vi "AUTON_Index.vi"(0 "Auton Array":dbl[][](array[numeric]), 5 "MeasuredHeading":dbl, 7 "LeftEncoder":dbl, 9 "RightEncoder":dbl) -> (4 "Right Drive":dbl, 6 "Left Drive":dbl, 8 "Harvester":dbl, 10 "Winch":dbl, 15 "Cam":dbl)   [LabVIEW 2013]
uses:
  Robot Global Data.vi
panel:
  in  "BallOnShooter":bool
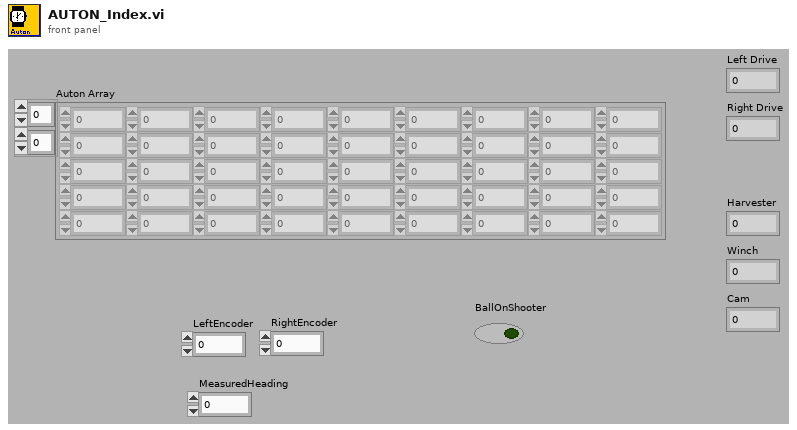
[diagram p1: front panel]
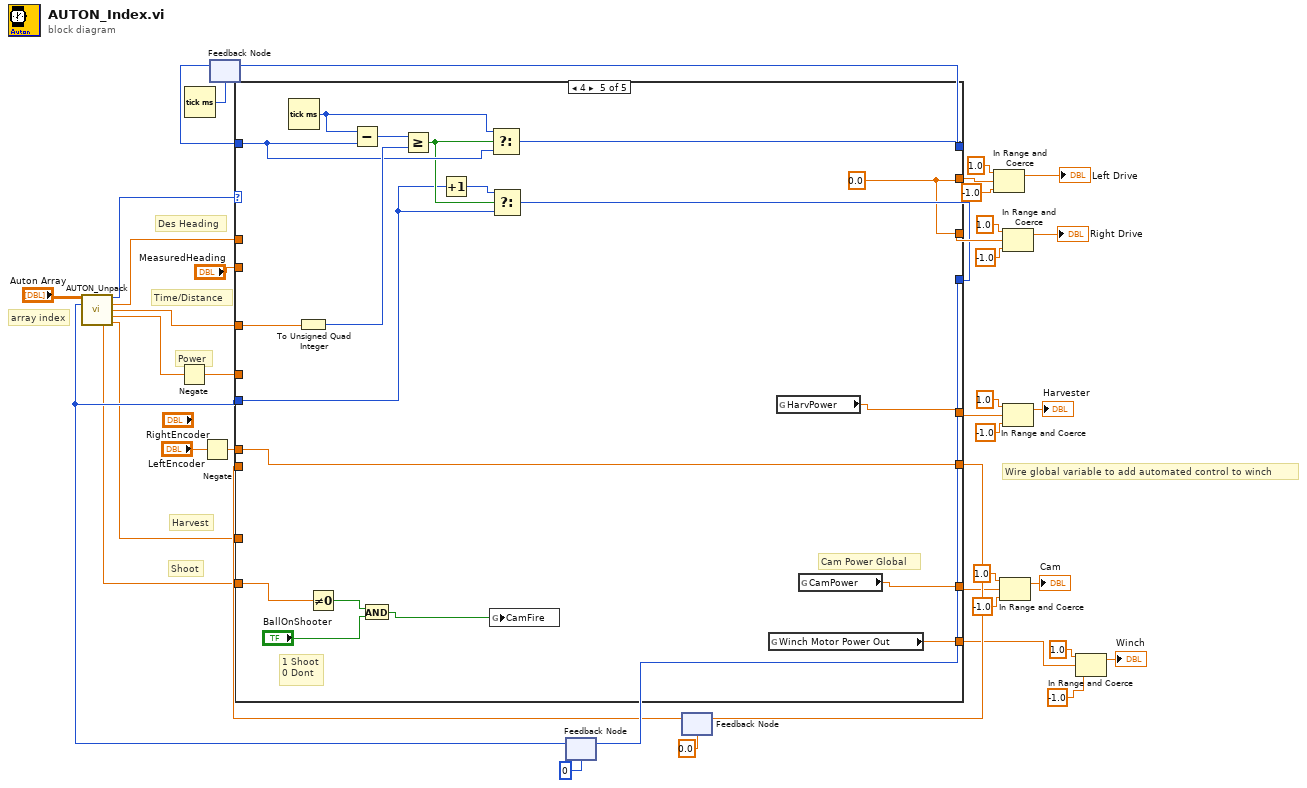
[diagram p0: block diagram]
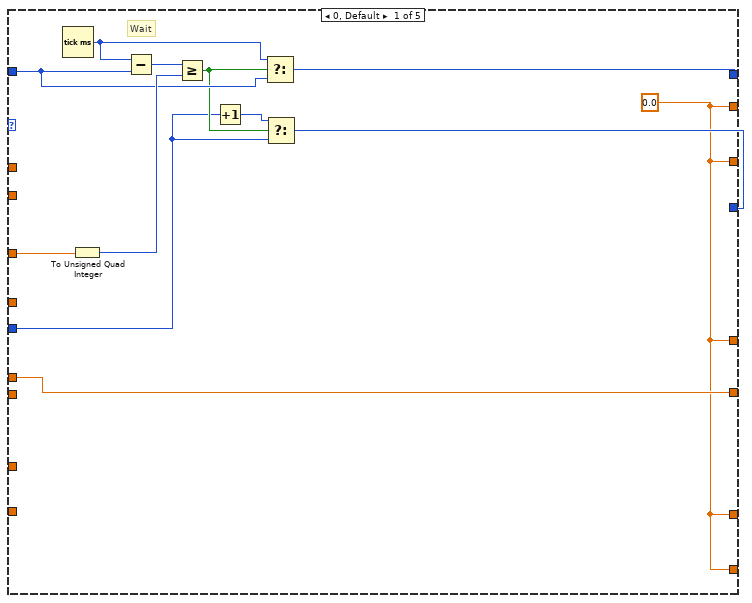
[diagram p2: hidden frame]
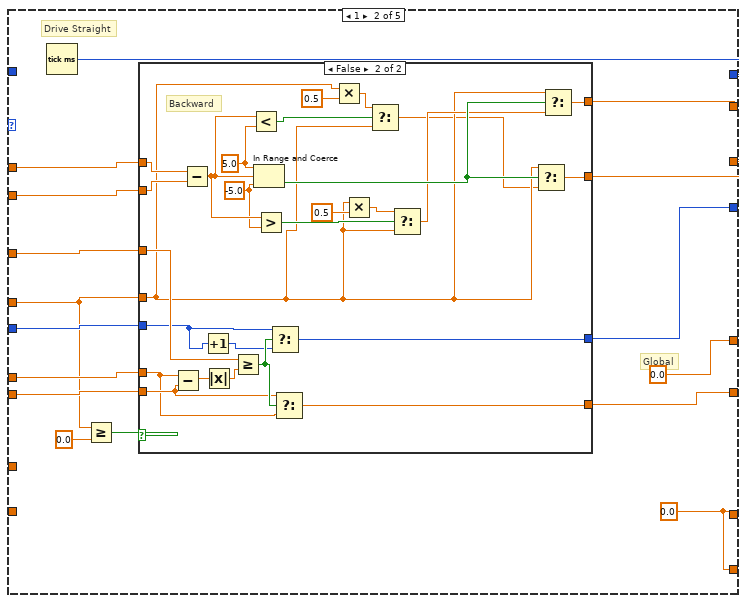
[diagram p3: hidden frame]
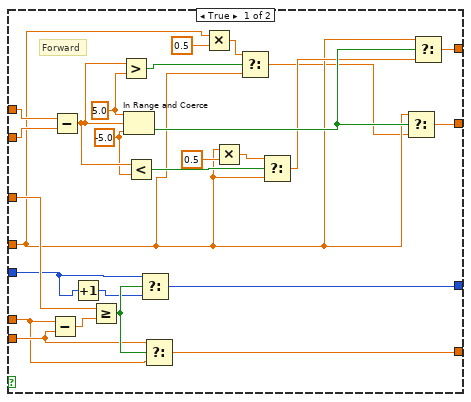
[diagram p4: hidden frame]
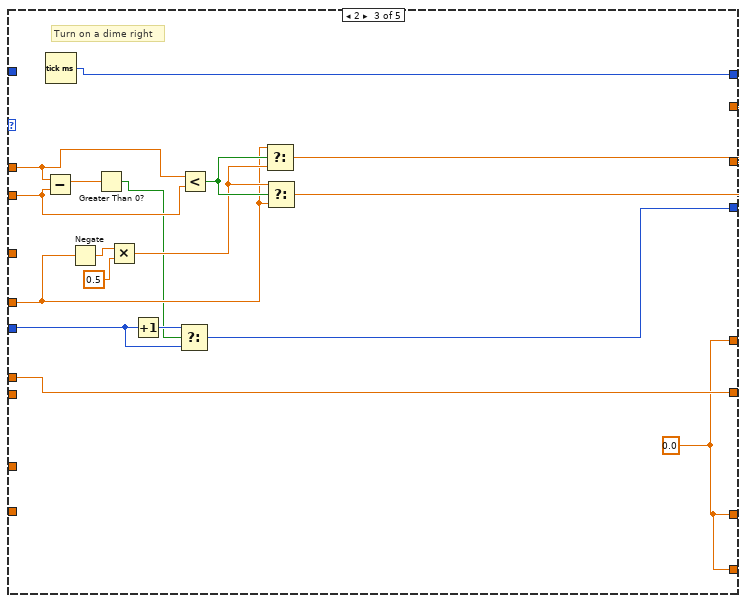
[diagram p5: hidden frame]
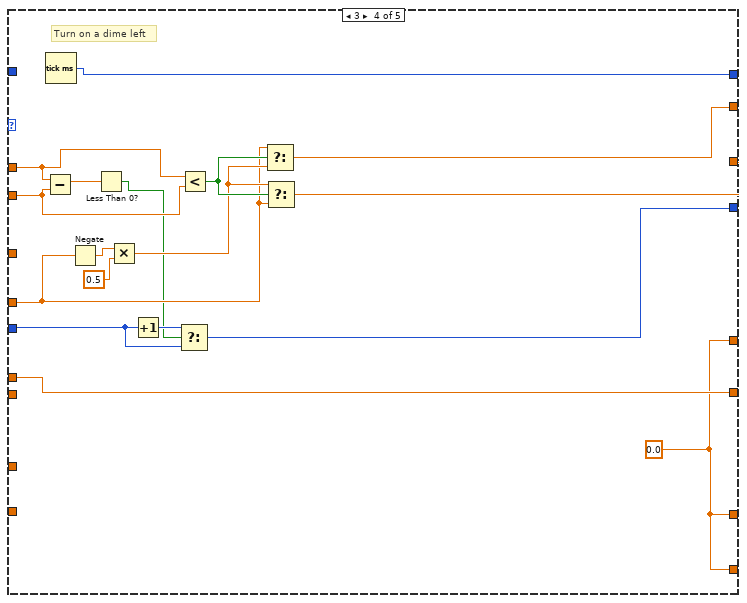
[diagram p6: hidden frame]
diagram:
  # "Shoot"
  # "Harvest"
  # "Wire global variable to add automated control to winch"
  # "Des Heading"
  # "Time/Distance"
  # "Power"
  # "array index"
  n1 = Tick Count (ms)() -> (millisecond timer value=w38:u32)
  n2 = Negate(x="LeftEncoder") -> (-x=w4:dbl)
  n3 = feedback #1(w38) -> (w39:u32)
  n4 = feedback #2(0) -> (w19:i32)
  n5 = call "AUTON_Unpack.vi"("all rows"="Auton Array", "Index"=w19) -> ("Primitive ID"=w22:i16, "Desired Heading"=w21:dbl, "Time/Distance"=w20:dbl, "Power"=w7:dbl, "Shoot"=w2:dbl, "Harvest"=w3:dbl)  [unwired: 8 in]
  n6 = Negate(x=w7) -> (-x=w6:dbl)
  n7 = feedback #3(0.0) -> (w24:dbl)
  n8 = case shown="4" w22 {
    tunnel: [w44 w66 w133 w150 w166] -> w26
    tunnel: w19 -> [w45 w61 w136 w153 w167]
    tunnel: [w52 w58 w138 w155 w174] -> w28
    tunnel: w39 -> [w49 _ _ _ w171]
    tunnel: w20 -> [w43 w67 _ _ w165]
    tunnel: w21 -> [_ w65 w131 w148 _]
    tunnel: [w41 w63 w134 w151 w164] -> w36
    tunnel: [w41 w62 w135 w152 w164] -> w29
    tunnel: w6 -> [_ w57 w125 w142 _]
    tunnel: w4 -> [w42 w59 w132 w149 w163]
    tunnel: "MeasuredHeading" -> [_ w64 w130 w147 _]
    tunnel: w24 -> [_ w60 _ _ _]
    tunnel: [w42 w68 w132 w149 w163] -> w23
    tunnel: [w41 w53 w122 w139 w161] -> w9
    tunnel: [w41 0.0 ("OutWheelF") w122 w139 w162] -> w8
    tunnel: w3 -> [_ _ _ _ _]
    tunnel: w2 -> [_ _ _ _ w160]
    tunnel: [w41 w53 w122 w139 w156] -> w1
    frame 0, Default {
      w41 = 0.0 ("Numeric")
      # "Wait"
      n9 = Tick Count (ms)() -> (millisecond timer value=w48:u32)
      n10 = To Unsigned Quad Integer(1:w43) -> (0:w50:u64)
      n11 = Subtract(x=w48, y=w49) -> (x-y=w51:u32)
      n12 = Greater Or Equal?(x=w51, y=w50) -> (x >= y?=w47:bool)
      n13 = Increment(x=w45) -> (x+1=w46:i32)
      n14 = Select(t=w48, s=w47, f=w49) -> (s? t:f=w52:u32)
      n15 = Select(t=w46, s=w47, f=w45) -> (s? t:f=w44:i32)
    }
    frame 1 {
      w53 = 0.0 ("OutWheelF")
      # "Global"
      # "Drive Straight"
      n16 = Tick Count (ms)() -> (millisecond timer value=w58:u32)
      n17 = Greater Or Equal?(x=w57, y=0.0) -> (x >= y?=w55:bool)
      n18 = case shown="False" w55 {
        tunnel: [w94 w121] -> w68
        tunnel: w67 -> [w92 w120]
        tunnel: [w90 w118] -> w66
        tunnel: w65 -> [w89 w117]
        tunnel: w64 -> [w88 w116]
        tunnel: [w86 w114] -> w63
        tunnel: [w85 w113] -> w62
        tunnel: w57 -> [w74 w102]
        tunnel: w61 -> [w71 w99]
        tunnel: w60 -> [w70 w98]
        tunnel: w59 -> [w69 w97]
        frame True {
          w82 = -5.0 ("lower limit")
          w84 = 5.0 ("upper limit")
          # "Forward"
          n19 = Subtract(x=w69, y=w70) -> (x-y=w93:dbl)
          n20 = Subtract(x=w89, y=w88) -> (x-y=w83:dbl)
          n21 = Increment(x=w71) -> (x+1=w72:i32)
          n22 = Greater Or Equal?(x=w92, y=w93) -> (x >= y?=w91:bool)
          n23 = Greater?(x=w83, y=w84) -> (0:w77:bool)
          n24 = In Range and Coerce(upper limit=w84, x=w83, lower limit=w82) -> (In Range?=w87:bool)  [unwired: 1 out]
          n25 = Less?(x=w83, y=w82) -> (x < y?=w81:bool)
          n26 = Select(t=w71, s=w91, f=w72) -> (s? t:f=w90:i32)
          n27 = Select(t=w70, s=w91, f=w69) -> (s? t:f=w94:dbl)
          n28 = Multiply(x=w74, y=0.5) -> (x*y=w76:dbl)
          n29 = Multiply(x=w74, y=0.5) -> (x*y=w79:dbl)
          n30 = Select(t=w76, s=w77, f=w74) -> (s? t:f=w73:dbl)
          n31 = Select(t=w79, s=w81, f=w74) -> (s? t:f=w78:dbl)
          n32 = Select(t=w74, s=w87, f=w73) -> (s? t:f=w85:dbl)
          n33 = Select(t=w74, s=w87, f=w78) -> (s? t:f=w86:dbl)
        }
        frame False {
          w110 = -5.0 ("lower limit")
          w112 = 5.0 ("upper limit")
          # "Backward"
          n34 = Subtract(x=w97, y=w98) -> (x-y=w95:dbl)
          n35 = Subtract(x=w117, y=w116) -> (x-y=w111:dbl)
          n36 = Increment(x=w99) -> (x+1=w100:i32)
          n37 = Absolute Value(x=w95) -> (abs(x)=w96:dbl)
          n38 = Greater Or Equal?(x=w120, y=w96) -> (x >= y?=w119:bool)
          n39 = Less?(x=w111, y=w112) -> (x < y?=w105:bool)
          n40 = In Range and Coerce(upper limit=w112, x=w111, lower limit=w110) -> (In Range?=w115:bool)  [unwired: 1 out]
          n41 = Greater?(x=w111, y=w110) -> (0:w109:bool)
          n42 = Select(t=w99, s=w119, f=w100) -> (s? t:f=w118:i32)
          n43 = Select(t=w98, s=w119, f=w97) -> (s? t:f=w121:dbl)
          n44 = Multiply(x=w102, y=0.5) -> (x*y=w104:dbl)
          n45 = Multiply(x=w102, y=0.5) -> (x*y=w107:dbl)
          n46 = Select(t=w104, s=w105, f=w102) -> (s? t:f=w101:dbl)
          n47 = Select(t=w107, s=w109, f=w102) -> (s? t:f=w106:dbl)
          n48 = Select(t=w102, s=w115, f=w101) -> (s? t:f=w113:dbl)
          n49 = Select(t=w102, s=w115, f=w106) -> (s? t:f=w114:dbl)
        }
      }
    }
    frame 2 {
      w122 = 0.0 ("Numeric")
      # "Turn on a dime right"
      n50 = Subtract(x=w131, y=w130) -> (x-y=w124:dbl)
      n51 = Tick Count (ms)() -> (millisecond timer value=w138:u32)
      n52 = Negate(x=w125) -> (-x=w128:dbl)
      n53 = Greater Than 0?(x=w124) -> (x > 0?=w123:bool)
      n54 = Multiply(x=w128, y=0.5) -> (x*y=w126:dbl)
      n55 = Increment(x=w136) -> (x+1=w137:i32)
      n56 = Select(t=w137, s=w123, f=w136) -> (s? t:f=w133:i32)
      n57 = Less?(x=w131, y=w130) -> (x < y?=w129:bool)
      n58 = Select(t=w125, s=w129, f=w126) -> (s? t:f=w134:dbl)
      n59 = Select(t=w126, s=w129, f=w125) -> (s? t:f=w135:dbl)
    }
    frame 3 {
      w139 = 0.0 ("Numeric")
      # "Turn on a dime left"
      n60 = Subtract(x=w148, y=w147) -> (x-y=w141:dbl)
      n61 = Tick Count (ms)() -> (millisecond timer value=w155:u32)
      n62 = Negate(x=w142) -> (-x=w145:dbl)
      n63 = Less Than 0?(x=w141) -> (x < 0?=w140:bool)
      n64 = Multiply(x=w145, y=0.5) -> (x*y=w143:dbl)
      n65 = Increment(x=w153) -> (x+1=w154:i32)
      n66 = Select(t=w154, s=w140, f=w153) -> (s? t:f=w150:i32)
      n67 = Less?(x=w148, y=w147) -> (x < y?=w146:bool)
      n68 = Select(t=w142, s=w146, f=w143) -> (s? t:f=w151:dbl)
      n69 = Select(t=w143, s=w146, f=w142) -> (s? t:f=w152:dbl)
    }
    frame 4 {
      w164 = 0.0 ("Numeric")
      # "1 Shoot\n0 Dont"
      # "Cam Power Global"
      n70 = Tick Count (ms)() -> (millisecond timer value=w170:u32)
      n71 = To Unsigned Quad Integer(1:w165) -> (0:w172:u64)
      n72 = Not Equal To 0?(x=w160) -> (x != 0?=w159:bool)
      n73 = Subtract(x=w170, y=w171) -> (x-y=w173:u32)
      n74 = And(x=w159, y="BallOnShooter") -> (x .and. y?=w157:bool)
      n75 = Greater Or Equal?(x=w173, y=w172) -> (x >= y?=w169:bool)
      n76 = Increment(x=w167) -> (x+1=w168:i32)
      n77 = global write "Robot Global Data.vi" "CamFire"(w157) -> ()
      n78 = Select(t=w170, s=w169, f=w171) -> (s? t:f=w174:u32)
      n79 = Select(t=w168, s=w169, f=w167) -> (s? t:f=w166:i32)
      n80 = global read "Robot Global Data.vi" "Winch Motor Power Out"() -> (w156:dbl)
      n81 = global read "Robot Global Data.vi" "HarvPower"() -> (w162:dbl)
      n82 = global read "Robot Global Data.vi" "CamPower"() -> (w161:dbl)
    }
  }
  n83 = feedback-in #1(w28) -> ()
  n84 = feedback-in #2(w26) -> ()
  n85 = feedback-in #3(w23) -> ()
  n86 = In Range and Coerce(upper limit=1.0, x=w36, lower limit=-1.0) -> (coerced(x)=→"Left Drive":dbl)  [unwired: 1 out]
  n87 = In Range and Coerce(upper limit=1.0, x=w9, lower limit=-1.0) -> (coerced(x)=→"Cam":dbl)  [unwired: 1 out]
  n88 = In Range and Coerce(upper limit=1.0, x=w29, lower limit=-1.0) -> (coerced(x)=→"Right Drive":dbl)  [unwired: 1 out]
  n89 = In Range and Coerce(upper limit=1.0, x=w8, lower limit=-1.0) -> (coerced(x)=→"Harvester":dbl)  [unwired: 1 out]
  n90 = In Range and Coerce(upper limit=1.0, x=w1, lower limit=-1.0) -> (coerced(x)=→"Winch":dbl)  [unwired: 1 out]
